vi "S2C_Shared_Proc_GetRefs.vi"(8 "Error In":errorcluster, 10 "Refs":string[][](array[string]), 11 "Label":string) -> (0 "Error Out":errorcluster, 3 "Reference":string)   [LabVIEW 2024]
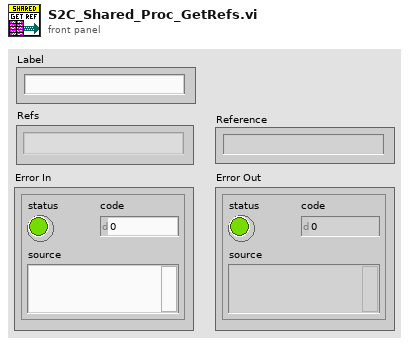
[diagram p1: front panel]
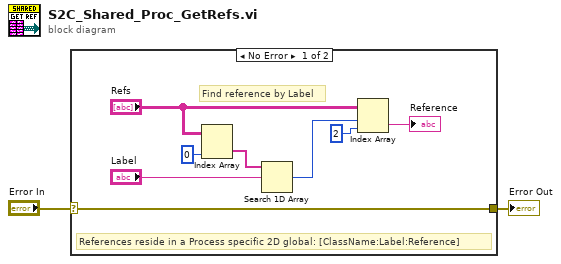
[diagram p0: block diagram]
diagram:
  n1 = case shown="No Error" "Error In" {
    selector: "Error In" -> [w4 w11]
    tunnel: [w4 w11] -> w1
    frame No Error {
      # "References reside in a Process specific 2D global: [ClassName:Label:Reference]"
      # "Find reference by Label"
      n2 = Index Array(array="Refs", index (col)=0 ("disabled index (col)")) -> (element=w9:string[])  [unwired: 1 in]
      n3 = Search 1D Array(1D array=w9, element="Label") -> (index of element=w7:i32)  [unwired: 1 in]
      n4 = Index Array(array="Refs", index (row)=w7, index (col)=2 ("disabled index (col)")) -> (element=→"Reference":string)
    }
    frame Error {
    }
  }
  "Error Out" <- w1
